vi "Actor Core.vi"(8 "error in":errorcluster, 11 "MFC in":refnum<class "MFC.lvclass">) -> (0 "error out":errorcluster, 3 "Actor out":refnum<class "Actor.lvclass">)   [LabVIEW 2018, in "MFC Actor.lvlib" / "MFC.lvclass"]
doc: "The user interface for this panel.\n\n----\nPlease see the following web address for additional documentation and tutorial information:\nhttp://www.mooregoodideas.com/mgi-panel-manager/\n\nAuthor: Derek Trepanier\n\nCopyright (c) 2018, Moore Good Ideas, Inc.\n\nAll rights reserved.\n\nRedistribution and use in source and binary forms, with or without modification, are permitted provided that the following conditions are met:\n\n * Redistributions of source code must retain the above copyright notice, this list of conditions and the following disclaimer.\n * Redistributions in binary form must reproduce the above copyright notice, this list of conditions and the following disclaimer in the documentation and/or other materials provided with the distribution.\n * Neither the name of Moore Good Ideas, Inc. nor the names of its contributors may be used to endorse or promote products derived from this software without specific prior written permission.\n\nTHIS SOFTWARE IS PROVIDED BY THE COPYRIGHT HOLDERS AND CONTRIBUTORS \"AS IS\" AND ANY EXPRESS OR IMPLIED WARRANTIES, INCLUDING, BUT NOT LIMITED TO, THE IMPLIED WARRANTIES OF MERCHANTABILITY AND FITNESS FOR A PARTICULAR PURPOSE ARE DISCLAIMED. IN NO EVENT SHALL THE COPYRIGHT OWNER OR CONTRIBUTORS BE LIABLE FOR ANY DIRECT, INDIRECT, INCIDENTAL, SPECIAL, EXEMPLARY, OR CONSEQUENTIAL DAMAGES (INCLUDING, BUT NOT LIMITED TO, PROCUREMENT OF SUBSTITUTE GOODS OR SERVICES; LOSS OF USE, DATA, OR PROFITS; OR BUSINESS INTERRUPTION) HOWEVER CAUSED AND ON ANY THEORY OF LIABILITY, WHETHER IN CONTRACT, STRICT LIABILITY, OR TORT (INCLUDING NEGLIGENCE OR OTHERWISE) ARISING IN ANY WAY OUT OF THE USE OF THIS SOFTWARE, EVEN IF ADVISED OF THE POSSIBILITY OF SUCH DAMAGE."
uses:
  MFC.lvclass
  C:/Program Files (x86)/National Instruments/LabVIEW 2018/vi.lib/MGI/Panel Manager/Panel Actor/Panel Actor/Panel Actor.lvclass
  C:/Program Files (x86)/National Instruments/LabVIEW 2018/vi.lib/ActorFramework/Actor/Actor.lvclass
  <vilib>/ActorFramework/Actor/Actor.lvclass
  MFC.lvclass/MFC.ctl
  <vilib>/ActorFramework/Actor/Actor.lvclass/Actor.ctl
  <vilib>/ActorFramework/Message Enqueuer/Message Enqueuer.lvclass/Message Enqueuer.ctl
  MFC Messages/Change Setpoint Msg/Change Setpoint Msg.lvclass/Change Setpoint Msg.ctl
  <vilib>/ActorFramework/Message Enqueuer/Init from Existing Queue.vi
  <vilib>/ActorFramework/Message Enqueuer/Enqueue.vi
  MFC Messages/Change Setpoint Msg/Change Setpoint Msg.lvclass
  C:/Program Files (x86)/National Instruments/LabVIEW 2018/vi.lib/ActorFramework/Message/Message.lvclass
  <vilib>/ActorFramework/Message Priority Queue/Priority Enqueue.vi
  <vilib>/ActorFramework/Message Enqueuer/Message Enqueuer.lvclass
  <vilib>/MGI/Panel Manager/Panel Actor/Panel Actor/Panel Actor.lvclass
  <instrlib>/Sierra Instruments Smart-Trak 100 Series/Sierra Instruments Smart-Trak 100 Series.lvlib
  ADM/Main.lvlib
panel:
  out "Flow":dbl
  in  "Setpoint":dbl
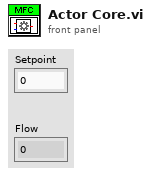
[diagram p1: front panel]
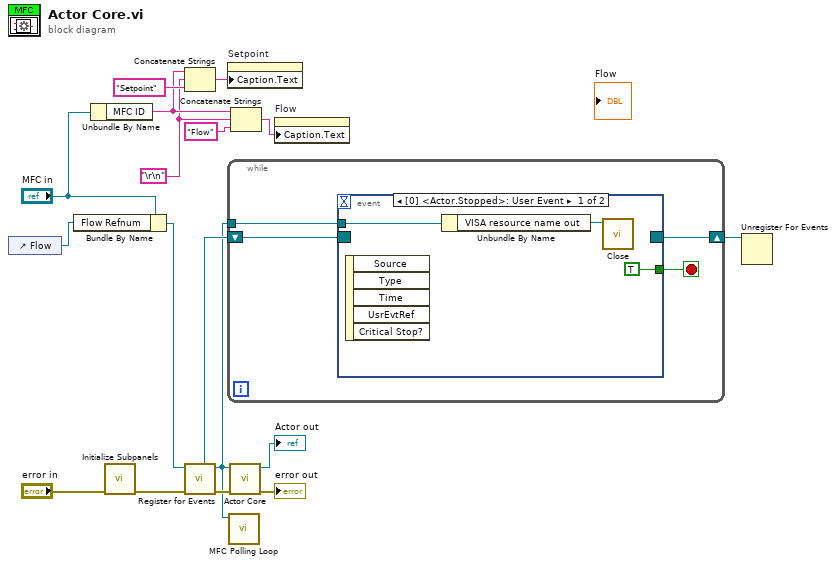
[diagram p0: block diagram]
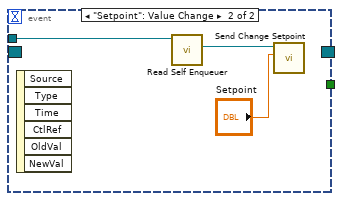
[diagram p2: hidden frame]
diagram:
  w9 = "\r\n"
  n1 = control-ref of="Flow"() -> (w6:refnum<vi>)
  n2 = Bundle By Name(cluster="MFC in", "Flow Refnum"=w6) -> (w2:refnum<class "MFC.lvclass">)
  n3 = Unbundle By Name("MFC in") -> ("MFC ID"=w10:string)
  n4 = call "Initialize Subpanels.vi"("error in (no error)"="error in") -> ("error out"=w5:errorcluster)  [unwired: 10 in]
  n5 = Concatenate Strings(w10, w9, "Setpoint") -> (w12:string)
  n6 = call <vilib>:"Register for Events.vi"("Error In"=w5, "Panel Actor in"=w2) -> ("Error Out"=w4:errorcluster, "Panel Actor out"=w1:refnum<class "MFC.lvclass">, "Pnl Actor"=w3:refnum<event-registration>)  [unwired: 6 in, 1 out]
  n7 = property on="Setpoint" class="DigNum (strict)"("Caption.Text"=w12) -> ()  [unwired: 2 in, 2 out]
  n8 = while {
    tunnel: w1 -> [w20]
    shift-right: [w19] -> w15
    shift-left: w3 -> [w18]
    stop <- w21 stop-if-true
    n9 = event shown="[0] <Actor.Stopped>: User Event" {
      selector: w18 -> [_ _]
      dyn-events: [_ _] -> w19
      timeout: _ -> [_ _]
      tunnel: [TRUE _] -> w21
      tunnel: w20 -> [w23 w26]
      event User Event {
        n10 = event-data() -> ()  [unwired: 1 in, 5 out]
        n11 = Unbundle By Name(w23) -> ("VISA resource name out"=w22:refnum<visa-resource-name>)
        n12 = call <instrlib>:"Close.vi"("VISA resource name"=w22) -> ()  [unwired: 10 in, 1 out]
      }
      event "Setpoint": Value Change {
        n13 = event-data() -> ()  [unwired: 1 in, 6 out]
        n14 = call <vilib>:"Read Self Enqueuer.vi"("Actor"=w26) -> ("Self Enqueuer"=w25:refnum<class "Message Enqueuer.lvclass">)  [unwired: 10 in]
        n15 = call "Send Change Setpoint.vi"("Setpoint"="Setpoint", "Message Enqueuer"=w25) -> ()  [unwired: 8 in, 2 out]
      }
    }
  }
  n16 = call "MFC Polling Loop.vi"("MFC Actor.lvlib:MFC.lvclass"=w1) -> ()  [unwired: 11 in]
  n17 = call-parent "Actor Core.vi"("error in"=w4, "Panel Actor in"=w1) -> ("error out"=→"error out":errorcluster, "Actor out"=→"Actor out":refnum<class "Actor.lvclass">)  [unwired: 8 in]
  n18 = Concatenate Strings(w10, w9, "Flow") -> (w11:string)
  n19 = property on="Flow" class="DigNum (strict)"("Caption.Text"=w11) -> ()  [unwired: 2 in, 2 out]
  n20 = Unregister For Events(event registration refnum=w15) -> ()  [unwired: 1 in, 1 out]
